vi "Error Cleanup.vi"(8 "error in (no error)":errorcluster, 11 "UDP in":refnum<class "UDP.lvclass">) -> (0 "error out":errorcluster, 3 "UDP out":refnum<class "UDP.lvclass">)   [LabVIEW 2019, in "Localhost Protocols.lvlib" / "UDP.lvclass"]
uses:
  UDP.lvclass
  UDP.lvclass/UDP.ctl
  Data Access/Read UDP Ref.vi
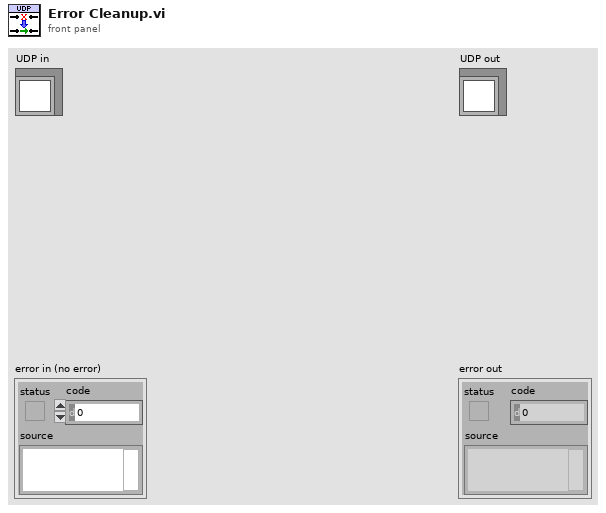
[diagram p1: front panel]
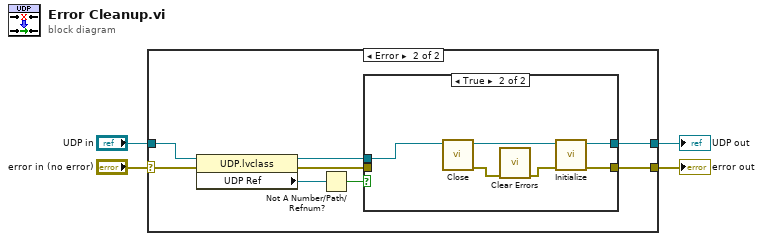
[diagram p0: block diagram]
diagram:
  n1 = case shown="Error" "error in (no error)" {
    selector: "error in (no error)" -> [w6 w13]
    tunnel: "UDP in" -> [w5 w14]
    tunnel: [w6 w8] -> w2
    tunnel: [w5 w7] -> w1
    frame No Error {
    }
    frame Error {
      n2 = property class="UDP.lvclass"(reference=w14, error in=w13) -> (reference out=w10:refnum<class "UDP.lvclass">, error out=w9:errorcluster, "UDP Ref"=w12:refnum<k16>)
      n3 = Not A Number/Path/Refnum?(number/path/refnum=w12) -> (NaN/Path/Refnum?=w11:bool)
      n4 = case shown="True" w11 {
        tunnel: w10 -> [w15 w20]
        tunnel: w9 -> [w16 _]
        tunnel: [w16 w22] -> w8
        tunnel: [w15 w21] -> w7
        frame False {
        }
        frame True {
          n5 = call-dynamic "Close.vi"("UDP in"=w20) -> ("error out"=w17:errorcluster, "UDP out"=w19:refnum<class "UDP.lvclass">)  [unwired: 9 in]
          n6 = call <vilib>:"Clear Errors.vi"("error in (no error)"=w17) -> ("error out"=w18:errorcluster)  [unwired: 5 in, 1 out]
          n7 = call-dynamic "Initialize.vi"("error in (no error)"=w18, "UDP in"=w19) -> ("error out"=w22:errorcluster, "UDP out"=w21:refnum<class "UDP.lvclass">)  [unwired: 8 in]
        }
      }
    }
  }
  "error out" <- w2
  "UDP out" <- w1
